vi "ContourPlot multi-channel v1.6.vi"() -> ()   [LabVIEW 2021]
uses:
  <vilib>/Utility/file.llb/Read Delimited Spreadsheet (DBL).vi
  <vilib>/gmath/NI_Gmath.lvlib
  <vilib>/Analysis/NI_AALPro.lvlib
panel:
  out "Channel number":i32=4
  out "Ready?":bool=TRUE
  in  "Tab Control":enum32{"Contour"}(tab)
  out "Intensity Graph":dbl[][](graph)
  in  "Begin":i32
  in  "x label index":i32
  in  "y label index":i32=1
  in  "intensisty plot channel index":i32=2
  in  "y cut x index":i32=1
  in  "length":i32=1001
  out "Y cut plot":cluster{dbl[], "Best Polynomial Fit":dbl[]}[](graph)
  out "Contour":cluster{dbl[], "Intensity Graph":dbl[]}(graph)={[-5.0, -5.2, -5.4, -5.6, -5.8, -6.0, -6.2, -6.4, -6.6, -6.8, -7.0, -7.2, -7.4, -7.6, -7.8, -8.0, -8.2, -8.4, -8.6, -8.8, -9.0, -9.2, -9.4, -9.6, -9.8, -10.0, -10.2, -10.4, -10.6, -10.8, -11.0, -11.2, -11.4, -11.6, -11.8, -12.0, -12.2, -12.4, -12.6, -12.8, -13.0, -13.2, -13.4, -13.6, -13.8, -14.0, -14.2, -14.4, -14.6, -14.8, -15.0, -15.2, -15.4, -15.6, -15.8, -16.0, -16.2, -16.4, -16.6, -16.8, -17.0, -17.2, -17.4, -17.6, -17.8, -18.0, -18.2, -18.4, -18.6, -18.8, -19.0, -19.2, -19.4, -19.6, -19.8, -20.0, -20.2, -20.4, -20.6, -20.8, -21.0, -21.2, -21.4, -21.6, -21.8, -22.0, -22.2, -22.4, -22.6, -22.8, -23.0, -23.2, -23.4, -23.6, -23.8, -24.0, -24.2, -24.4, -24.6, -24.8, -25.0, -25.2, -25.4, -25.6, -25.8, -26.0, -26.2, -26.4, -26.6, -26.8, -27.0, -27.2, -27.4, -27.6, -27.8, -28.0, -28.2, -28.4, -28.6, -28.8, -29.0, -29.2, -29.4, -29.6, -29.8, -30.0, -30.2, -30.4, -30.6, -30.8, -31.0, -31.2, -31.4, -31.6, -31.8, -32.0, -32.2, -32.4, -32.6, -32.8, -33.0, -33.2, -33.4, -33.6, -33.8, -34.0, -34.2, -34.4, -34.6, -34.8, -35.0], "Intensity Graph"=[4.86231805057675, 6.436293888828695, 8.591457398879687, 7.255398306956646, 5.876125466214011, 4.894715846199911, 5.869115183702168, 5.484295660421036, 5.412133037940738, 6.223369437488266, 6.01655113598483, 5.662872498810897, 5.939408303311771, 6.069376620294221, 5.918679391154276, 6.778633718020687, 5.778412549582421, 5.7423224226209095, 5.921011239363087, 5.654587541534491, 5.708715175223074, 5.955225574852862, 5.829384637229394, 5.364170470256028, 5.193034239024225, 11.69477770873895, 5.765579316238428, 6.630996921369482, 7.790700167511403, 5.868805656007415, 6.162611519662277, 6.067968278076005, 5.002169120518238, 5.929359861277952, 5.722168354487355, 5.642396420189638, 7.145100347878553, 6.039555545548941, 5.850671580170111, 5.971667449383636, 6.017984810475952, 8.902079322729222, 5.927124239412467, 5.952279581708947, 6.021556251691794, 5.801690237676107, 5.8599041411033115, 5.982199393819112, 5.887584529138133, 5.7114716996145845, 6.2351030591240075, 5.954727221773576, 5.841998391487643, 5.909147470907817, 6.745623220393876, 5.877770772668234, 5.888136399583406, 5.937602205347099, 5.4263532103479175, 5.743059178199999, 5.793773424862577, 5.873620039220291, 5.934875857371172, 5.874452743403241, 5.89668231838174, 5.7843202163255985, 5.862315116902885, 5.316154417154915, 5.930773034611936, 5.916453757175602, 5.661612421288643, 6.044778245912455, 6.002360836514385, 7.274149330907029, 5.773803959637983, 6.4864325106273, 5.928847187140029, 6.006597722161248, 5.567457214808729, 5.859542402076649, 5.8622721191508145, 6.029017433268589, 5.813966219902066, 5.945586693419107, 5.999954328777123, 5.755082152043619, 6.14894852708364, 5.938059638346117, 6.075816297085337, 6.783514503307689, 6.033612020938373, 7.701827757537912, 6.038944285921784, 5.966508067134863, 6.64722700189968, 5.811096232924369, 5.898350134655884, 5.561370167056399, 6.229958212948102, 5.933290858784923, 5.484337283463988, 5.8729420069163005, 6.843142020544011, 5.820023205793059, 5.900743983612079, 5.625652129020998, 5.887134683490854, 5.9067101898033485, 5.928738081719839, 6.005663919769562, 6.431696429180311, 5.398490362361453, 5.933517530670519, 5.796838682773862, 5.901759135599033, 5.883135682476253, 5.844709362539378, 5.9052473975889335, 5.885134386179859, 6.113003195289019, 5.951414683847996, 5.813362100989305, 5.75626066011884, 6.413980966048724, 5.940924287308521, 6.033977012397427, 6.07987166659468, 5.907234565573321, 5.903754853956933, 5.902113695120557, 5.351636508691941, 6.288029850411143, 4.476622549808645, 5.82614742914228, 5.745518914332306, 5.569317185745332, 5.993181305787751, 5.880690370351448, 5.885347644972266, 6.005236943892372, 5.872928785293299, 6.106436946623544, 5.88068934777971, 5.797938724557806, 5.877310204271547, 5.940497597465883, 5.864732105847283, 5.9594632573214135, 5.21335433305795, 5.889973180822589, 9.714360175378053]}
  in  "threshold":dbl=0.18 step=0.01
  in  "extract method":string(combo)="Raw Data"
  in  "Button":bool
  in  "book number":i32=1
  in  "file path (dialog if empty)":path=path "C:/Users/dvh-collab-user/Desktop/20230313 Robert sample"
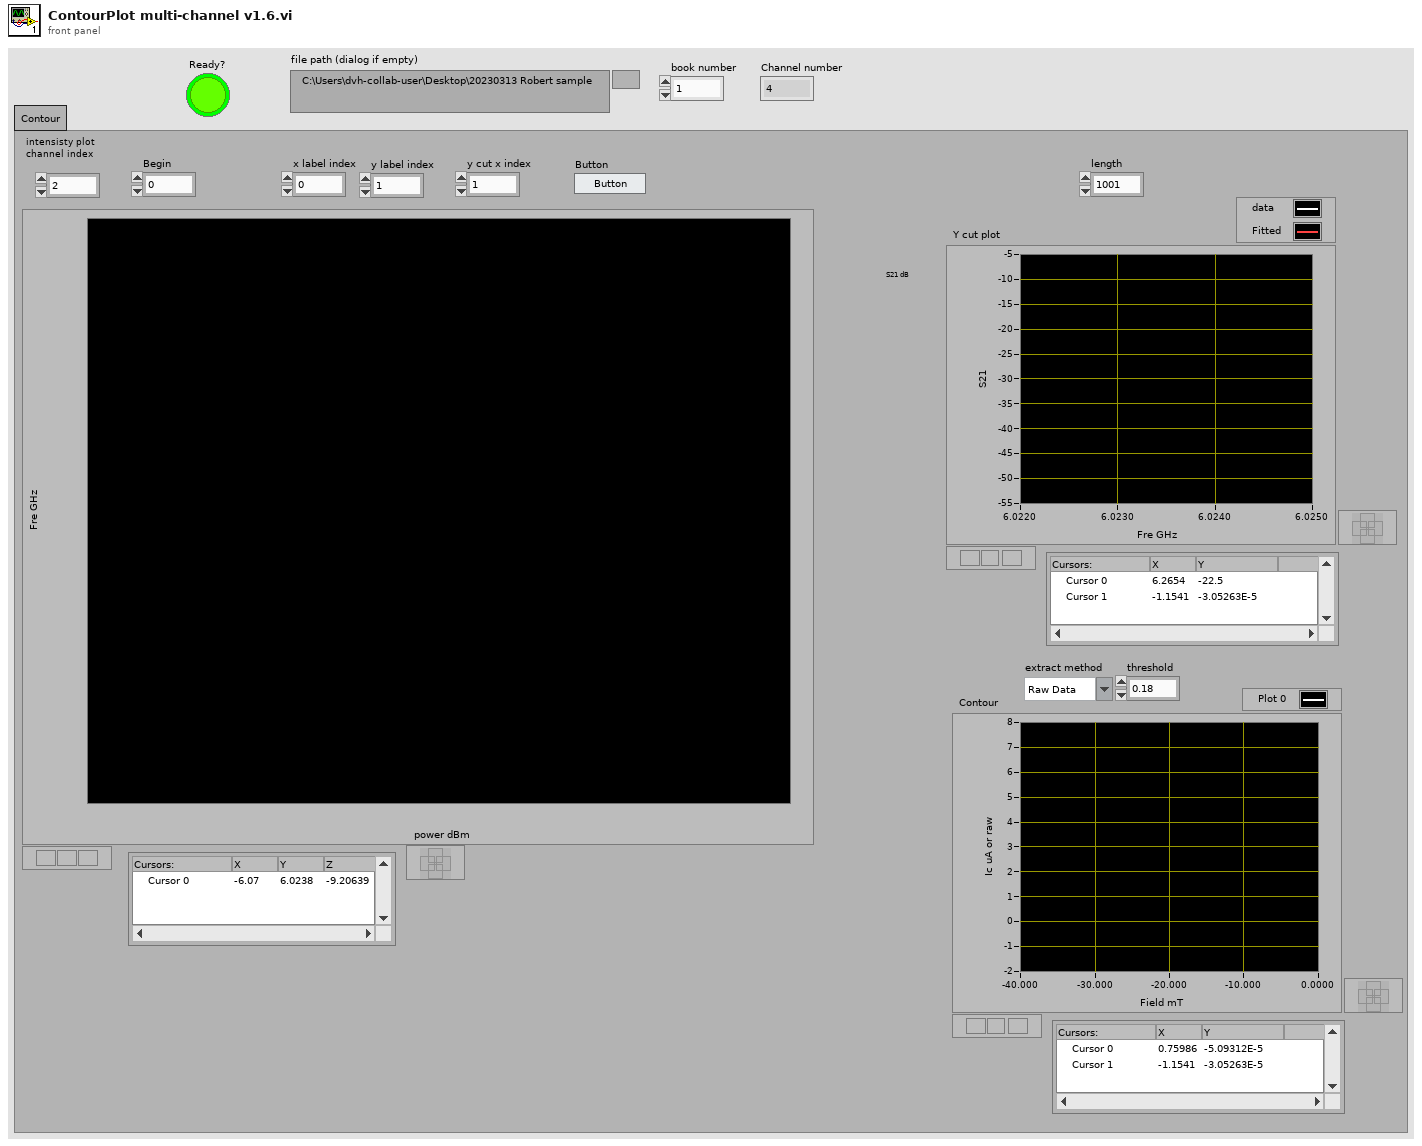
[diagram p1: front panel]
types:
  T1 = cluster{"all rows":dbl[], "Best Polynomial Fit":dbl[]}
  T2 = cluster{"all rows":dbl[], "Best Polynomial Fit":dbl[]}[]
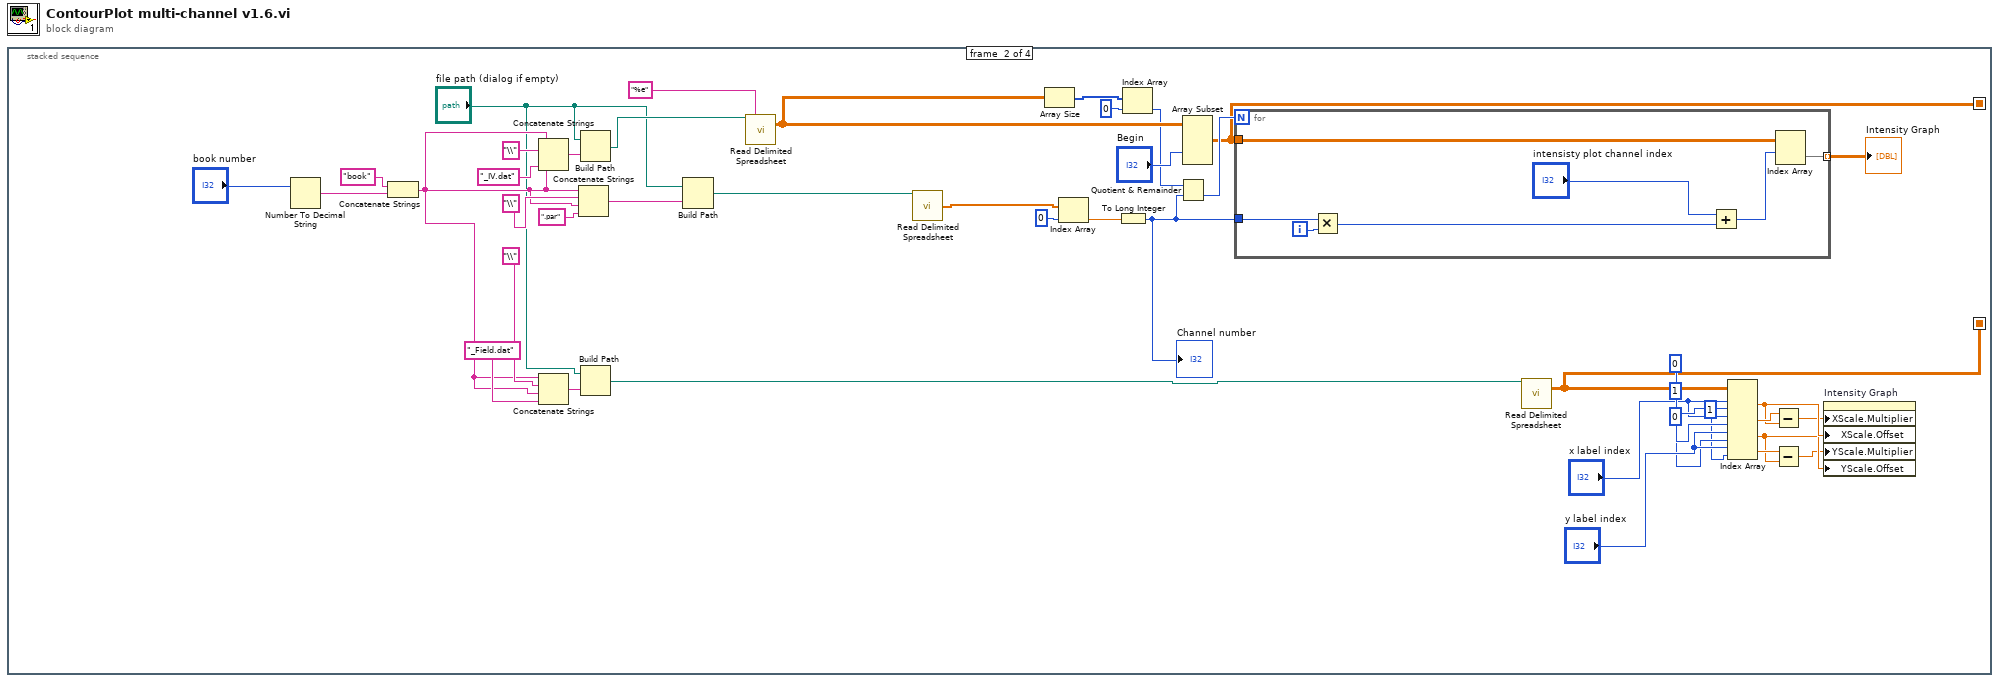
[diagram p0: block diagram]
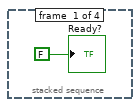
[diagram p2: hidden frame]
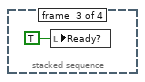
[diagram p3: hidden frame]
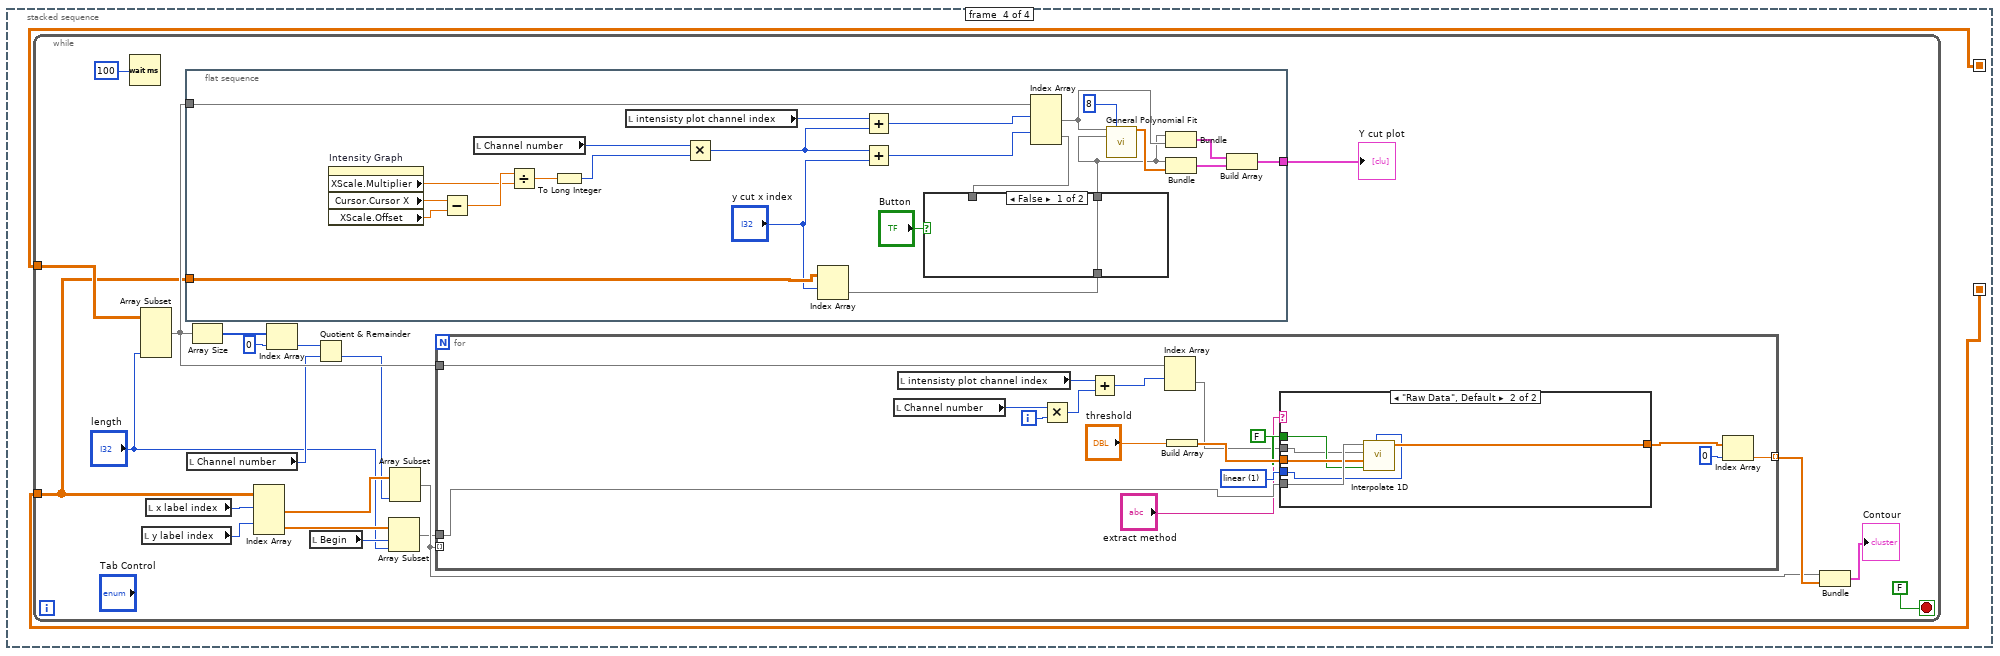
[diagram p4: hidden frame]
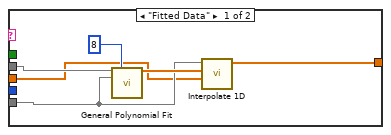
[diagram p5: hidden frame]
diagram:
  n1 = stacked-sequence {
    seq-local: [_ w3 _ _] -> [_ _ _ w54]
    seq-local: [_ w2 _ _] -> [_ _ _ w53]
    frame #0 {
      "Ready?" <- FALSE ("Ready?")
    }
    frame #1 {
      n2 = Number To Decimal String(number="book number") -> (decimal integer string=w40:string)  [unwired: 1 in]
      n3 = Concatenate Strings("book" ("string"), w40) -> (w29:string)
      n4 = Concatenate Strings(w29, "\\" ("string"), w29, "_IV.dat" ("string")) -> (w41:string)
      n5 = Concatenate Strings(w29, "\\" ("string"), w29, "_Field.dat" ("string")) -> (w23:string)
      n6 = Concatenate Strings(w29, "\\" ("string"), w29, ".par" ("string")) -> (w42:string)
      n7 = Build Path(base path="file path (dialog if empty)", name or relative path=w41) -> (appended path=w44:path)
      n8 = Build Path(base path="file path (dialog if empty)", name or relative path=w23) -> (appended path=w16:path)
      n9 = Build Path(base path="file path (dialog if empty)", name or relative path=w42) -> (appended path=w43:path)
      n10 = call-poly <vilib>:"Read Delimited Spreadsheet.vi"("file path (dialog if empty)"=w44, "format (%.3f)"="%e") -> ("all rows"=w26:dbl[][])  [unwired: 8 in, 5 out]
      n11 = call-poly <vilib>:"Read Delimited Spreadsheet.vi"("file path (dialog if empty)"=w43) -> ("first row"=w22:dbl[])  [unwired: 9 in, 5 out]
      n12 = Array Size(array=w26) -> (size(s)=w34:i32[])
      n13 = Index Array(array=w22, index=0) -> (element=w20:dbl)
      n14 = To Long Integer(number=w20) -> (32bit integer=w18:i32)
      "Channel number" <- w18
      n15 = Index Array(array=w34, index=0) -> (element=w19:i32)
      n16 = Quotient & Remainder(x=w19, y=w18) -> (floor(x/y)=w17:i32)  [unwired: 1 out]
      n17 = Array Subset(array=w26, index (col)="Begin") -> (w3:dbl[][])  [unwired: 3 in]
      n18 = for {
        N: w17 -> [_]
        tunnel: w3 -> [w50]
        tunnel: [w49] -> w27 mode=indexing
        tunnel: w18 -> [w46]
        i -> [w51]
        n19 = Multiply(x=w46, y=w51) -> (x*y=w45:i32)
        n20 = Add(x="intensisty plot channel index", y=w45) -> (x+y=w48:i32)
        n21 = Index Array(array=w50, index (row)=w48) -> (element=w49:dbl[])  [unwired: 1 in]
      }
      "Intensity Graph" <- w27
      n22 = call-poly <vilib>:"Read Delimited Spreadsheet.vi"("file path (dialog if empty)"=w16) -> ("all rows"=w2:dbl[][])  [unwired: 9 in, 5 out]
      n23 = Index Array(array=w2, index (row) #1="x label index", index (col) #1=0 ("disabled index (col)"), index (row) #2="x label index", index (col) #2=1 ("disabled index (col)"), index (row) #3="y label index", index (col) #3=0 ("disabled index (col)"), index (row) #4="y label index", index (col) #4=1 ("disabled index (col)")) -> (element #1=w11:dbl, element #2=w12:dbl, element #3=w5:dbl, element #4=w6:dbl)
      n24 = Subtract(x=w12, y=w11) -> (x-y=w10:dbl)
      n25 = Subtract(x=w6, y=w5) -> (x-y=w4:dbl)
      n26 = property on="Intensity Graph" class="IntGraph (strict)"("XScale.Multiplier"=w10, "XScale.Offset"=w11, "YScale.Multiplier"=w4, "YScale.Offset"=w5) -> ()  [unwired: 2 in, 2 out]
    }
    frame #2 {
      n27 = local write "Ready?"(TRUE ("Ready?")) -> ()
    }
    frame #3 {
      n28 = while {
        tunnel: w53 -> [w55]
        tunnel: w54 -> [w68]
        stop <- FALSE stop-if-true
        n29 = Wait (ms)(milliseconds to wait=u32 100) -> ()  [unwired: 1 out]
        n30 = Array Subset(array=w68, length (col)="length") -> (w67:dbl[][])  [unwired: 3 in]
        n31 = local read "y label index"() -> (w70:i32)
        n32 = local read "x label index"() -> (w69:i32)
        n33 = flat-sequence {
          tunnel: [w110] -> w75
          tunnel: w67 -> [w122]
          tunnel: w55 -> [w106]
          frame #0 {
            n34 = property on="Intensity Graph" class="IntGraph (strict)"() -> ("XScale.Multiplier"=w126:dbl, "Cursor.Cursor X"=w125:dbl, "XScale.Offset"=w124:dbl)  [unwired: 2 in, 2 out]
            n35 = Subtract(x=w125, y=w124) -> (x-y=w127:dbl)
            n36 = local read "Channel number"() -> (w120:i32)
            n37 = Divide(x=w127, y=w126) -> (x/y=w123:dbl)
            n38 = To Long Integer(number=w123) -> (32bit integer=w121:i32)
            n39 = local read "intensisty plot channel index"() -> (w118:i32)
            n40 = Multiply(x=w120, y=w121) -> (x*y=w119:i32)
            n41 = Index Array(array=w106, index (row)="y cut x index") -> (element=w104:dbl[])  [unwired: 1 in]
            n42 = Add(x=w118, y=w119) -> (x+y=w117:i32)
            n43 = Add(x=w119, y="y cut x index") -> (x+y=w116:i32)
            n44 = Index Array(array=w122, index (row) #1=w117, index (row) #2=w116) -> (element #1=w115:dbl[], element #2=w108:dbl[])  [unwired: 2 in]
            n45 = case shown="False" "Button" {
              tunnel: w108 -> [_ w129]
              tunnel: [w128 w129] -> w107
              tunnel: w104 -> [w128 _]
              frame False {
              }
              frame True {
              }
            }
            n46 = call <vilib>:"General Polynomial Fit.vi"("Y"=w115, "polynomial order"=8, "X"=w107) -> ("Best Polynomial Fit"=w113:dbl[])  [unwired: 9 in, 3 out]
            n47 = Bundle("all rows"=w107, w115) -> (w112:cluster{"all rows":dbl[], dbl[]})  [unwired: 1 in]
            n48 = Bundle("all rows"=w107, "Best Polynomial Fit"=w113) -> (w111:T1)  [unwired: 1 in]
            n49 = Build Array(w112, w111) -> (w110:T2)
          }
        }
        n50 = local read "Channel number"() -> (w63:i32)
        n51 = Array Size(array=w67) -> (size(s)=w66:i32[])
        n52 = Index Array(array=w55, index (row) #1=w69, index (row) #2=w70) -> (element #1=w62:dbl[], element #2=w59:dbl[])  [unwired: 2 in]
        n53 = Index Array(array=w66, index=0) -> (element=w64:i32)
        n54 = local read "Begin"() -> (w58:i32)
        n55 = Quotient & Remainder(x=w64, y=w63) -> (floor(x/y)=w61:i32)  [unwired: 1 out]
        n56 = Array Subset(array=w59, index=w58, length="length") -> (w56:dbl[])
        n57 = Array Subset(array=w62, length=w61) -> (w60:dbl[])  [unwired: 1 in]
        n58 = for {
          tunnel: w67 -> [w91]
          tunnel: w56 -> [w87]
          tunnel: [w88] -> w71 mode=indexing
          tunnel: w60 -> [_] mode=indexing
          i -> [w90]
          w83 = 1 items=["nearest", "linear", "spline", "cubic Hermite", "Lagrange"] ("method")
          n59 = local read "Channel number"() -> (w81:i32)
          n60 = local read "intensisty plot channel index"() -> (w79:i32)
          n61 = Multiply(x=w81, y=w90) -> (x*y=w80:i32)
          n62 = Add(x=w79, y=w80) -> (x+y=w78:i32)
          n63 = Index Array(array=w91, index (row)=w78) -> (element=w77:dbl[])  [unwired: 1 in]
          n64 = Build Array("threshold") -> (w84:dbl[])
          n65 = case shown="\"Raw Data\", Default" "extract method" {
            tunnel: w87 -> [w94 w103]
            tunnel: [w92 w102] -> w86
            tunnel: w84 -> [w93 w101]
            tunnel: w83 -> [_ w100]
            tunnel: FALSE ("X is monotonic") -> [_ w99]
            tunnel: w77 -> [w97 w98]
            frame "Fitted Data" {
              n66 = call <vilib>:"General Polynomial Fit.vi"("Y"=w97, "polynomial order"=8, "X"=w94) -> ("Best Polynomial Fit"=w95:dbl[])  [unwired: 9 in, 3 out]
              n67 = call <vilib>:"Interpolate 1D.vi"("xi"=w93, "X"=w95, "Y"=w94) -> ("yi"=w92:dbl[])  [unwired: 6 in, 2 out]
            }
            frame "Raw Data", Default {
              n68 = call <vilib>:"Interpolate 1D.vi"("method"=w100, "X is monotonic"=w99, "xi"=w101, "X"=w98, "Y"=w103) -> ("yi"=w102:dbl[])  [unwired: 4 in, 2 out]
            }
          }
          n69 = Index Array(array=w86, index=0) -> (element=w88:dbl)
        }
        n70 = Bundle(w60, w71) -> (→"Contour":cluster{dbl[], dbl[]})  [unwired: 1 in]
        "Y cut plot" <- w75
      }
    }
  }
